vi "Test_In_Range_ARGB_Image.vi"(8 "error in (no error)":errorcluster, 11 "Test Case In":refnum<class "Image.lvclass">) -> (0 "error out":errorcluster, 3 "Test Case Out":refnum<class "Image.lvclass">)   [LabVIEW 2020, in "g_ar_toolkit.test.lvlib" / "Image.lvclass"]
uses:
  Image.lvclass
  Image.lvclass/Image.ctl
  g_ar_toolkit.image/g_ar_toolkit.image.lvlib
  g_ar_toolkit.image/Image Size (Fixed).ctl
  g_ar_toolkit.image/CreateEmptyImageGreyscale.vi
  g_ar_toolkit.image/In-Range Image Colour Range.ctl
  4993e8ee-a06a-463a-9684-69129f64d5ce.vi
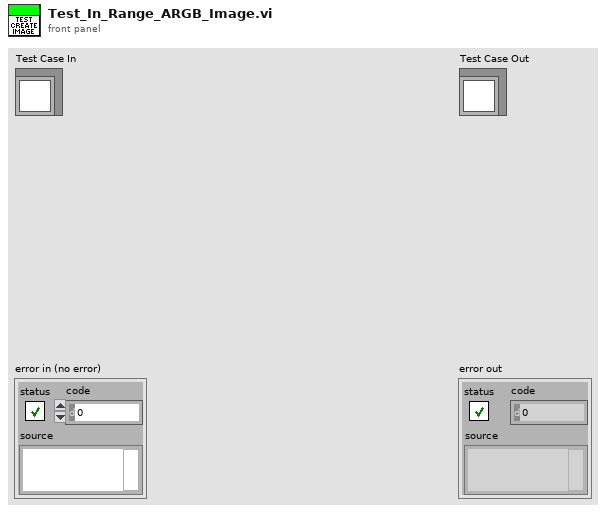
[diagram p1: front panel]
types:
  T1 = typedef "g_ar_toolkit.image.lvlib/In-Range Image Colour Range.ctl" = cluster{"Lower":u32, "Upper":u32}
  T2 = typedef "g_ar_toolkit.image.lvlib/Image Size (Fixed).ctl" = cluster{"Width":u16, "Height":u16}
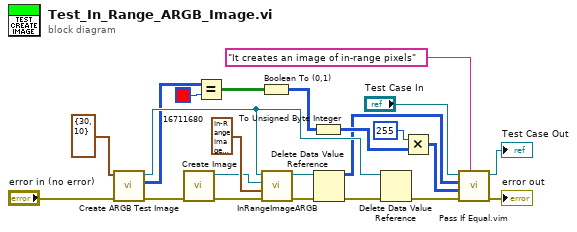
[diagram p0: block diagram]
diagram:
  n1 = call "Create ARGB Test Image.vi"("error in (no error)"="error in (no error)", "Preallocated Image Size"=T2 {"Width"=30, "Height"=10} ("Preallocated Image Size (Default - 0,0)")) -> ("error out"=w18:errorcluster, "24-bit pixmap"=w9:u32[][], "Data Value Reference out"=w10:refnum<data-value>)  [unwired: 7 in]
  n2 = call-poly "Create Image.vi"("error in (no error)"=w18) -> ("error out"=w17:errorcluster, "New Greyscale Image"=w11:refnum<data-value>)  [unwired: 9 in]
  n3 = Equal?(x=w9, y=u32 16711680 ("color(black)")) -> (x = y?=w7:bool[][])
  n4 = Boolean To (0,1)(Boolean=w7) -> (0, 1=w6:i16[][])
  n5 = call "InRangeImageARGB.vi"("error in (no error)"=w17, "In-Range Image Colour Range"=T1 {"Lower"=16711680, "Upper"=16760576}, "In-Range-Result"=w11, "ARGB Image Source"=w10) -> ("error out"=w12:errorcluster, "In-Range-Result (duplicate)"=w1:refnum<data-value>)  [unwired: 6 in]
  n6 = To Unsigned Byte Integer(number=w6) -> (unsigned 8bit integer=w5:u8[][])
  n7 = Delete Data Value Reference(data value reference=w1, error in=w12) -> (data value=w2:u8[][], error out=w16:errorcluster)
  n8 = Delete Data Value Reference(data value reference=w10, error in=w16) -> (error out=w15:errorcluster)  [unwired: 1 out]
  n9 = Multiply(x=u8 255, y=w5) -> (x*y=w3:u8[][])
  n10 = call "Pass If Equal.vim"("Description"="It creates an image of in-range pixels", "error in (no error)"=w15, "Actual"=w3, "Expected"=w2, "LUnit Test Case In"="Test Case In") -> ("error out"=→"error out":errorcluster, "LUnit Test Case Out"=→"Test Case Out":refnum<class "Image.lvclass">)  [unwired: 5 in]
